vi "PulseDetect60withIndices.vi"(9 "Laser bits in":bool[](array[boolean])=[FALSE, FALSE, FALSE, FALSE, FALSE, FALSE, FALSE, FALSE, FALSE, FALSE], 10 "Last region":bool=TRUE, 11 "Last laser bit in":bool) -> (1 "Region array out":bool[](array[boolean]), 2 "New last region out":bool, 3 "New last laser bit out":bool)   [LabVIEW 2012]
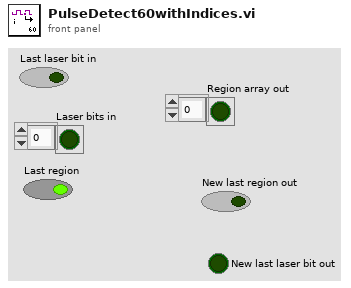
[diagram p1: front panel]
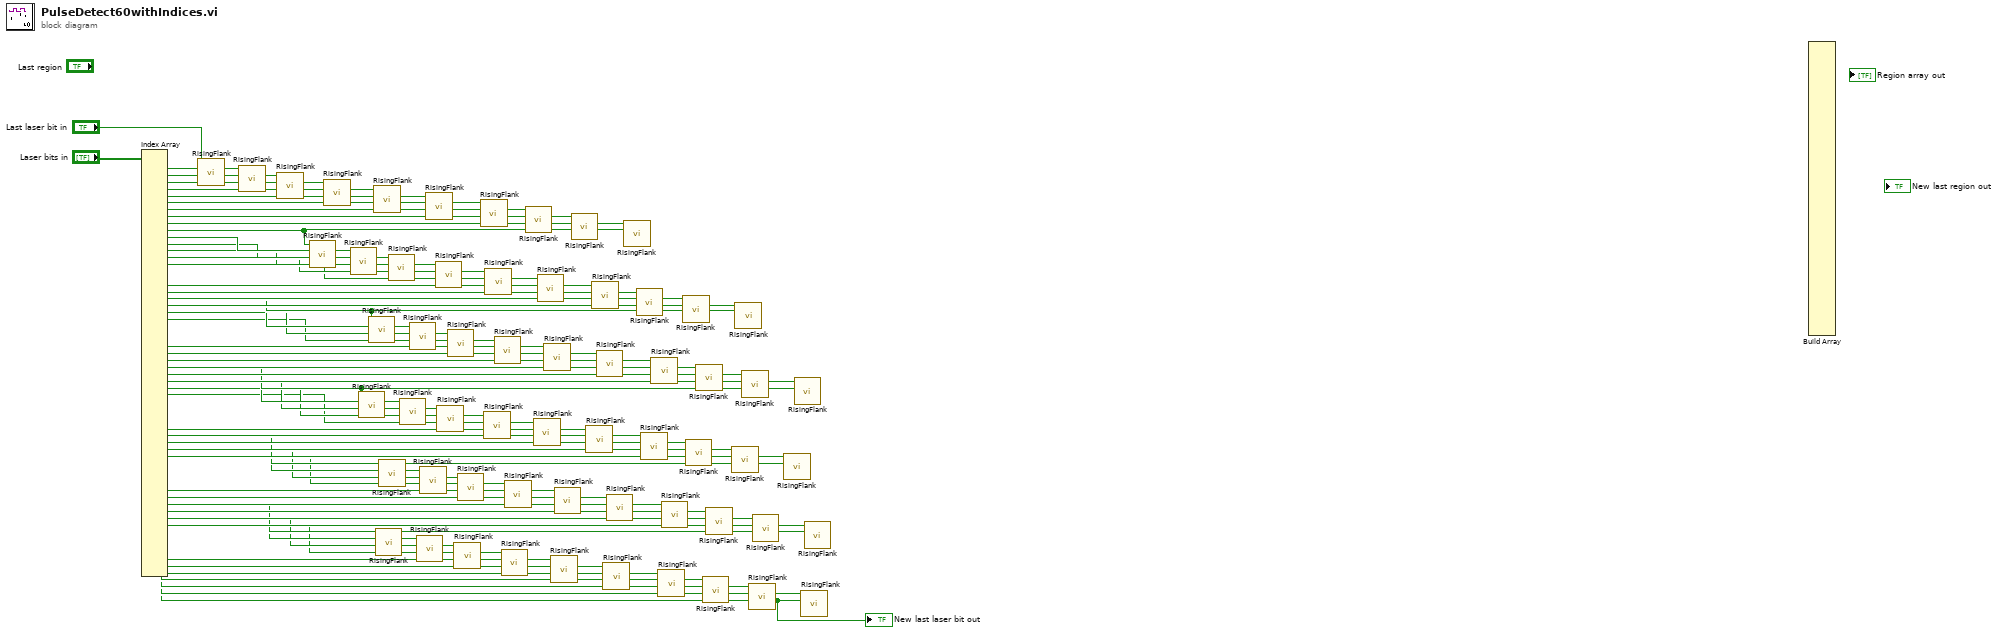
[diagram p0: block diagram]
diagram:
  n1 = Index Array(array="Laser bits in") -> (element #1=w60:bool, element #2=w59:bool, element #3=w58:bool, element #4=w57:bool, element #5=w56:bool, element #6=w55:bool, element #7=w54:bool, element #8=w53:bool, element #9=w52:bool, element #10=w51:bool, element #11=w50:bool, element #12=w49:bool, element #13=w48:bool, element #14=w47:bool, element #15=w46:bool, element #16=w45:bool, element #17=w44:bool, element #18=w43:bool, element #19=w42:bool, element #20=w41:bool, element #21=w40:bool, element #22=w39:bool, element #23=w38:bool, element #24=w37:bool, element #25=w36:bool, element #26=w35:bool, element #27=w34:bool, element #28=w33:bool, element #29=w32:bool, element #30=w31:bool, element #31=w30:bool, element #32=w29:bool, element #33=w28:bool, element #34=w27:bool, element #35=w26:bool, element #36=w25:bool, element #37=w24:bool, element #38=w23:bool, element #39=w22:bool, element #40=w21:bool, element #41=w20:bool, element #42=w19:bool, element #43=w18:bool, element #44=w17:bool, element #45=w16:bool, element #46=w15:bool, element #47=w14:bool, element #48=w13:bool, element #49=w12:bool, element #50=w11:bool, element #51=w10:bool, element #52=w9:bool, element #53=w8:bool, element #54=w7:bool, element #55=w6:bool, element #56=w5:bool, element #57=w4:bool, element #58=w3:bool, element #59=w2:bool, element #60=w1:bool)  [unwired: 60 in]
  "New last laser bit out" <- w1
  n2 = call "RisingFlank.vi"("2nd sample"=w60, "1st sample"="Last laser bit in") -> ()  [unwired: 7 in, 1 out]
  n3 = call "RisingFlank.vi"("2nd sample"=w59, "1st sample"=w60) -> ()  [unwired: 7 in, 1 out]
  n4 = call "RisingFlank.vi"("2nd sample"=w58, "1st sample"=w59) -> ()  [unwired: 7 in, 1 out]
  n5 = call "RisingFlank.vi"("2nd sample"=w50, "1st sample"=w51) -> ()  [unwired: 7 in, 1 out]
  n6 = call "RisingFlank.vi"("2nd sample"=w57, "1st sample"=w58) -> ()  [unwired: 7 in, 1 out]
  n7 = call "RisingFlank.vi"("2nd sample"=w49, "1st sample"=w50) -> ()  [unwired: 7 in, 1 out]
  n8 = call "RisingFlank.vi"("2nd sample"=w30, "1st sample"=w31) -> ()  [unwired: 7 in, 1 out]
  n9 = call "RisingFlank.vi"("2nd sample"=w40, "1st sample"=w41) -> ()  [unwired: 7 in, 1 out]
  n10 = call "RisingFlank.vi"("2nd sample"=w56, "1st sample"=w57) -> ()  [unwired: 7 in, 1 out]
  n11 = call "RisingFlank.vi"("2nd sample"=w10, "1st sample"=w11) -> ()  [unwired: 7 in, 1 out]
  n12 = call "RisingFlank.vi"("2nd sample"=w20, "1st sample"=w21) -> ()  [unwired: 7 in, 1 out]
  n13 = call "RisingFlank.vi"("2nd sample"=w48, "1st sample"=w49) -> ()  [unwired: 7 in, 1 out]
  n14 = call "RisingFlank.vi"("2nd sample"=w29, "1st sample"=w30) -> ()  [unwired: 7 in, 1 out]
  n15 = call "RisingFlank.vi"("2nd sample"=w39, "1st sample"=w40) -> ()  [unwired: 7 in, 1 out]
  n16 = call "RisingFlank.vi"("2nd sample"=w9, "1st sample"=w10) -> ()  [unwired: 7 in, 1 out]
  n17 = call "RisingFlank.vi"("2nd sample"=w19, "1st sample"=w20) -> ()  [unwired: 7 in, 1 out]
  n18 = call "RisingFlank.vi"("2nd sample"=w55, "1st sample"=w56) -> ()  [unwired: 7 in, 1 out]
  n19 = call "RisingFlank.vi"("2nd sample"=w47, "1st sample"=w48) -> ()  [unwired: 7 in, 1 out]
  n20 = call "RisingFlank.vi"("2nd sample"=w28, "1st sample"=w29) -> ()  [unwired: 7 in, 1 out]
  n21 = call "RisingFlank.vi"("2nd sample"=w38, "1st sample"=w39) -> ()  [unwired: 7 in, 1 out]
  n22 = call "RisingFlank.vi"("2nd sample"=w8, "1st sample"=w9) -> ()  [unwired: 7 in, 1 out]
  n23 = call "RisingFlank.vi"("2nd sample"=w18, "1st sample"=w19) -> ()  [unwired: 7 in, 1 out]
  n24 = call "RisingFlank.vi"("2nd sample"=w54, "1st sample"=w55) -> ()  [unwired: 7 in, 1 out]
  n25 = call "RisingFlank.vi"("2nd sample"=w27, "1st sample"=w28) -> ()  [unwired: 7 in, 1 out]
  n26 = call "RisingFlank.vi"("2nd sample"=w46, "1st sample"=w47) -> ()  [unwired: 7 in, 1 out]
  n27 = call "RisingFlank.vi"("2nd sample"=w37, "1st sample"=w38) -> ()  [unwired: 7 in, 1 out]
  n28 = call "RisingFlank.vi"("2nd sample"=w7, "1st sample"=w8) -> ()  [unwired: 7 in, 1 out]
  n29 = call "RisingFlank.vi"("2nd sample"=w17, "1st sample"=w18) -> ()  [unwired: 7 in, 1 out]
  n30 = call "RisingFlank.vi"("2nd sample"=w53, "1st sample"=w54) -> ()  [unwired: 7 in, 1 out]
  n31 = call "RisingFlank.vi"("2nd sample"=w26, "1st sample"=w27) -> ()  [unwired: 7 in, 1 out]
  n32 = call "RisingFlank.vi"("2nd sample"=w45, "1st sample"=w46) -> ()  [unwired: 7 in, 1 out]
  n33 = call "RisingFlank.vi"("2nd sample"=w36, "1st sample"=w37) -> ()  [unwired: 7 in, 1 out]
  n34 = call "RisingFlank.vi"("2nd sample"=w6, "1st sample"=w7) -> ()  [unwired: 7 in, 1 out]
  n35 = call "RisingFlank.vi"("2nd sample"=w16, "1st sample"=w17) -> ()  [unwired: 7 in, 1 out]
  n36 = call "RisingFlank.vi"("2nd sample"=w52, "1st sample"=w53) -> ()  [unwired: 7 in, 1 out]
  n37 = call "RisingFlank.vi"("2nd sample"=w25, "1st sample"=w26) -> ()  [unwired: 7 in, 1 out]
  n38 = call "RisingFlank.vi"("2nd sample"=w44, "1st sample"=w45) -> ()  [unwired: 7 in, 1 out]
  n39 = call "RisingFlank.vi"("2nd sample"=w35, "1st sample"=w36) -> ()  [unwired: 7 in, 1 out]
  n40 = call "RisingFlank.vi"("2nd sample"=w5, "1st sample"=w6) -> ()  [unwired: 7 in, 1 out]
  n41 = call "RisingFlank.vi"("2nd sample"=w15, "1st sample"=w16) -> ()  [unwired: 7 in, 1 out]
  n42 = call "RisingFlank.vi"("2nd sample"=w51, "1st sample"=w52) -> ()  [unwired: 7 in, 1 out]
  n43 = call "RisingFlank.vi"("2nd sample"=w43, "1st sample"=w44) -> ()  [unwired: 7 in, 1 out]
  n44 = call "RisingFlank.vi"("2nd sample"=w24, "1st sample"=w25) -> ()  [unwired: 7 in, 1 out]
  n45 = call "RisingFlank.vi"("2nd sample"=w34, "1st sample"=w35) -> ()  [unwired: 7 in, 1 out]
  n46 = call "RisingFlank.vi"("2nd sample"=w4, "1st sample"=w5) -> ()  [unwired: 7 in, 1 out]
  n47 = call "RisingFlank.vi"("2nd sample"=w14, "1st sample"=w15) -> ()  [unwired: 7 in, 1 out]
  n48 = call "RisingFlank.vi"("2nd sample"=w42, "1st sample"=w43) -> ()  [unwired: 7 in, 1 out]
  n49 = call "RisingFlank.vi"("2nd sample"=w23, "1st sample"=w24) -> ()  [unwired: 7 in, 1 out]
  n50 = call "RisingFlank.vi"("2nd sample"=w33, "1st sample"=w34) -> ()  [unwired: 7 in, 1 out]
  n51 = call "RisingFlank.vi"("2nd sample"=w3, "1st sample"=w4) -> ()  [unwired: 7 in, 1 out]
  n52 = call "RisingFlank.vi"("2nd sample"=w13, "1st sample"=w14) -> ()  [unwired: 7 in, 1 out]
  n53 = call "RisingFlank.vi"("2nd sample"=w22, "1st sample"=w23) -> ()  [unwired: 7 in, 1 out]
  n54 = call "RisingFlank.vi"("2nd sample"=w41, "1st sample"=w42) -> ()  [unwired: 7 in, 1 out]
  n55 = call "RisingFlank.vi"("2nd sample"=w32, "1st sample"=w33) -> ()  [unwired: 7 in, 1 out]
  n56 = call "RisingFlank.vi"("2nd sample"=w2, "1st sample"=w3) -> ()  [unwired: 7 in, 1 out]
  n57 = call "RisingFlank.vi"("2nd sample"=w12, "1st sample"=w13) -> ()  [unwired: 7 in, 1 out]
  n58 = call "RisingFlank.vi"("2nd sample"=w21, "1st sample"=w22) -> ()  [unwired: 7 in, 1 out]
  n59 = call "RisingFlank.vi"("2nd sample"=w31, "1st sample"=w32) -> ()  [unwired: 7 in, 1 out]
  n60 = call "RisingFlank.vi"("2nd sample"=w1, "1st sample"=w2) -> ()  [unwired: 7 in, 1 out]
  n61 = call "RisingFlank.vi"("2nd sample"=w11, "1st sample"=w12) -> ()  [unwired: 7 in, 1 out]
  n62 = Build Array() -> ()  [unwired: 43 in, 1 out]
